vi "4.convolution.vi"() -> ()   [LabVIEW 2018]
uses:
  <vilib>/Analysis/2dsp.llb/1D Convolution (DBL).vi
  <vilib>/measure/maspectr.llb/FFT Spectrum (Mag-Phase) for 1 Chan.vi
  <vilib>/measure/NI_MABase.lvlib
  <vilib>/Analysis/NI_AALPro.lvlib
  <vilib>/measure/NI_MAPro.lvlib
panel:
  in  "Stop Button":bool
  out "sinus signa  x(t)l":waveform(dbl)(graph)
  out "square signal h(t)":waveform(dbl)(graph)
  out "spectre of y(t)":cluster{"f0":dbl, "df":dbl, "magnitude":dbl[]}(graph)
  out "result of convolution":dbl[](graph)
  in  "frequency \n  of square sig":dbl=10.0 format="%0.2p"
  in  "frequency \n  of sinus sig":dbl=10.0 format="%0.2p"
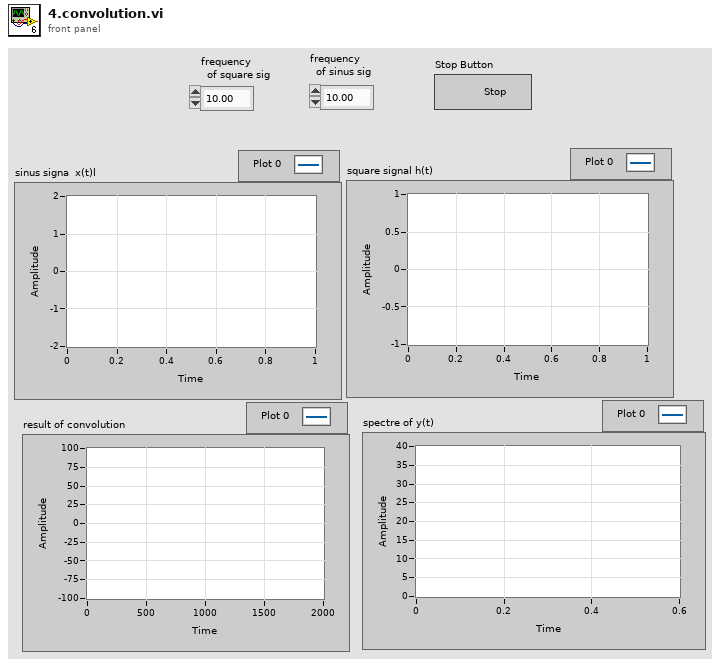
[diagram p1: front panel]
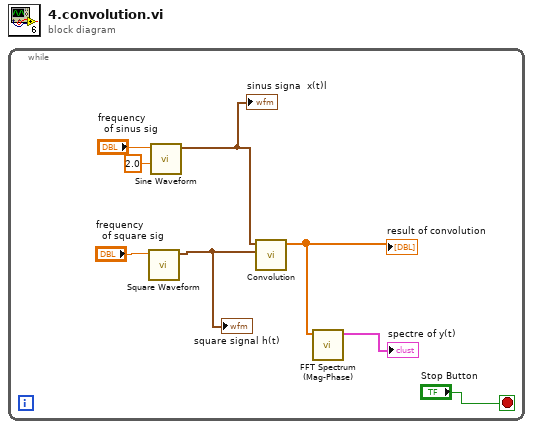
[diagram p0: block diagram]
diagram:
  n1 = while {
    stop <- "Stop Button" stop-if-true
    n2 = call <vilib>:"Square Waveform.vi"("frequency"="frequency \n  of square sig") -> ("signal out"=w3:waveform(dbl))  [unwired: 9 in, 1 out]
    "square signal h(t)" <- w3
    n3 = call <vilib>:"Sine Waveform.vi"("amplitude"=2.0, "frequency"="frequency \n  of sinus sig") -> ("signal out"=w2:waveform(dbl))  [unwired: 8 in, 1 out]
    "sinus signa  x(t)l" <- w2
    n4 = call-poly <vilib>:"Convolution.vi"("Y"=w3, "X"=w2) -> ("X * Y"=w6:dbl[])  [unwired: 8 in, 1 out]
    "result of convolution" <- w6
    n5 = call-poly <vilib>:"FFT Spectrum (Mag-Phase).vi"("time signal"=w6) -> ("magnitude"=→"spectre of y(t)":cluster{"f0":dbl, "df":dbl, "magnitude":dbl[]})  [unwired: 6 in, 4 out]
  }
